vi "FTW-ActorExtended-LaunchChildActor.vi"(0 "FTW Actor Connector Type":refnum<class "FTW-ActorExtended.lvclass">, 5 "Configuration":string="{\n  \"Identity\": \"ActorName\",\n  \"DebugEnableInboxLogging\": false,\n  \"DebugEnableJobLogging\": false,\n  \"InboxAddress\": \"inproc://*\",\n  \"DebugShowPanel\": false\n}", 7 "Actor VI Refnum":refnum<vi>, 9 "Timeout":i32=1000 format="%dmsec", 11 "error in":errorcluster) -> (4 "FTW-ActorExtended.lvclass":refnum<class "FTW-ActorExtended.lvclass">, 6 "Initialized Response":string, 8 "Instance Inbox Address":string, 15 "error out":errorcluster)   [LabVIEW 2013, in "FTW-ActorExtended.lvclass"]
doc: "This is the spawn new actor that was used for a while. It lacks the minimum strict inputs required to launch an actor."
uses:
  FTW-ActorExtended.lvclass
  Connector/FTW-ActorConnector.lvclass
  JSON/FTW-JSON-Core-LibraryError.vi
  Error/FTW-ERR-NoErrorConstant.vi
  JSON/FTW-JSON-Core-LibraryFilepath.vi
  Reflection/FTW-Reflection-Type.vi
  Error/FTW-ERR-ThrowError.vi
  Error/FTW-ERR-ThrowGenericError.vi
  JSON/FTW-JSON-Core-GetFlattenedValue.vi
  CodeGen/JSON Deserialize/FTW-JSON-Deserialize.xnode
  JSON/FTW-JSON-Native-GetFlattenedValue.vi
  JSON/FTW-JSON-Validate.vi
panel:
  # "Inputs"
  # "Outputs"
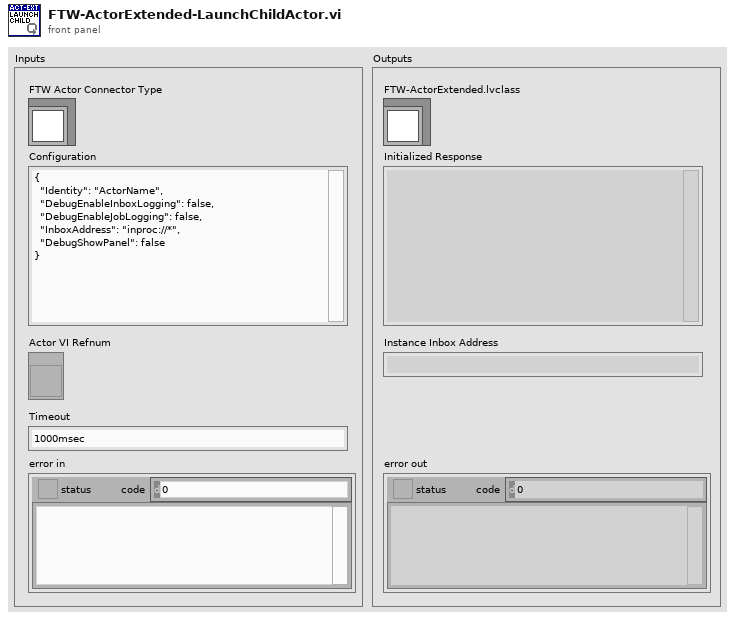
[diagram p1: front panel]
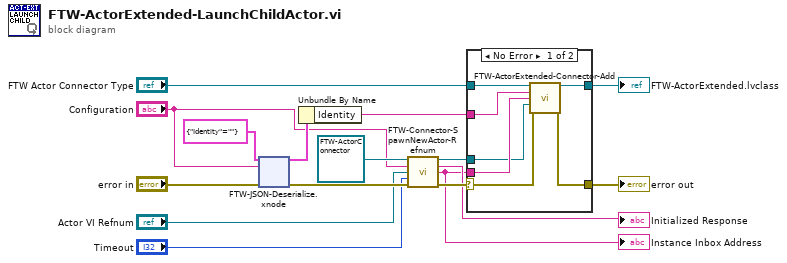
[diagram p0: block diagram]
diagram:
  n1 = xnode "FTW-JSON-Deserialize.xnode"("Type and Defaults"=cluster{"Identity":string} {"Identity"=""}, "JSON String"="Configuration", "error in"="error in") -> ("Values"=w15:cluster{"Identity":string}, "error out"=w13:errorcluster)
  n2 = Unbundle By Name(w15) -> ("Identity"=w11:string)
  n3 = call "FTW-Connector-SpawnNewActor-Refnum.vi"("FTW Actor Connector Type"=refnum<class "FTW-ActorConnector.lvclass"> refnum, "Configuration"="Configuration", "Actor VI Refnum"="Actor VI Refnum", "Timeout"="Timeout", "error in"=w13) -> ("FTW Actor Connector"=w10:refnum<class "FTW-ActorConnector.lvclass">, "Initialized Response"=→"Initialized Response":string, "Instance Inbox Address"=w4:string, "error out"=w12:errorcluster)  [unwired: 7 in]
  "Instance Inbox Address" <- w4
  n4 = case shown="No Error" w12 {
    selector: w12 -> [w23 w24]
    tunnel: "FTW Actor Connector Type" -> [w21 w25]
    tunnel: [w20 w25] -> w6
    tunnel: [w22 w24] -> w3
    tunnel: w11 -> [w19 _]
    tunnel: w4 -> [w18 _]
    tunnel: w10 -> [w17 _]
    frame No Error {
      n5 = call "FTW-ActorExtended-Connector-Add.vi"("FTW-ActorExtended In"=w21, "Identity"=w19, "Inbox Address"=w18, "Connection"=w17, "error in"=w23) -> ("FTW-ActorExtended Out"=w20:refnum<class "FTW-ActorExtended.lvclass">, "error out"=w22:errorcluster)  [unwired: 9 in]
    }
    frame Error {
    }
  }
  "error out" <- w3
  "FTW-ActorExtended.lvclass" <- w6
